vi "Get Flex Channel.vi"(11 "Element Type":variant) -> (3 "Data Type":variant)   [LabVIEW 2020, in "FlexBlock.xnode"]
uses:
  FlexBlock.xnode
  <resource>/ChannelSupport/_ChannelScriptingSupport/_ChannelScriptingSupport.lvlib
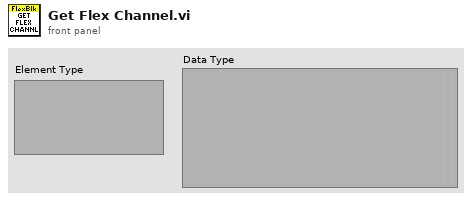
[diagram p1: front panel]
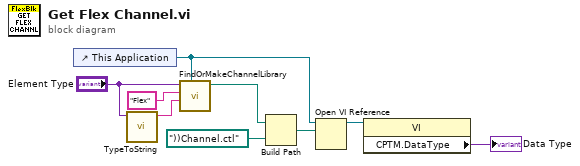
[diagram p0: block diagram]
diagram:
  n1 = control-ref of="This Application"() -> (w1:refnum<vi>)
  n2 = call <resource>:"TypeToString.vi"("type"="Element Type") -> ("string"=w8:string)  [unwired: 10 in]
  n3 = call <resource>:"FindOrMakeChannelLibrary.vi"("app"=w1, "typestring"=w8, "class"="Flex", "elt type"="Element Type") -> ("channel folder"=w6:path)  [unwired: 6 in, 1 out]
  n4 = Build Path(base path=w6, name or relative path=path "))Channel.ctl") -> (appended path=w4:path)
  n5 = Open VI Reference(application reference (local)=w1, vi path=w4) -> (vi reference=w3:refnum<vi>)  [unwired: 4 in, 1 out]
  n6 = property class="VI"(reference=w3) -> ("CPTM.DataType"=→"Data Type":variant)  [unwired: 1 in, 2 out]
